vi "QR Reader.vi"() -> (0 "3":bool, 1 "2":bool, 2 "1":bool)   [LabVIEW 2017]
uses:
  <vilib>/vision/NI_Vision_Development_Module.lvlib
panel:
  out "index1":string
  out "QR_array":string[](array[string])
  out "Image Display":T1(plugin-control)
  in  "Stop (F)":bool
  out "Barcode Data":string
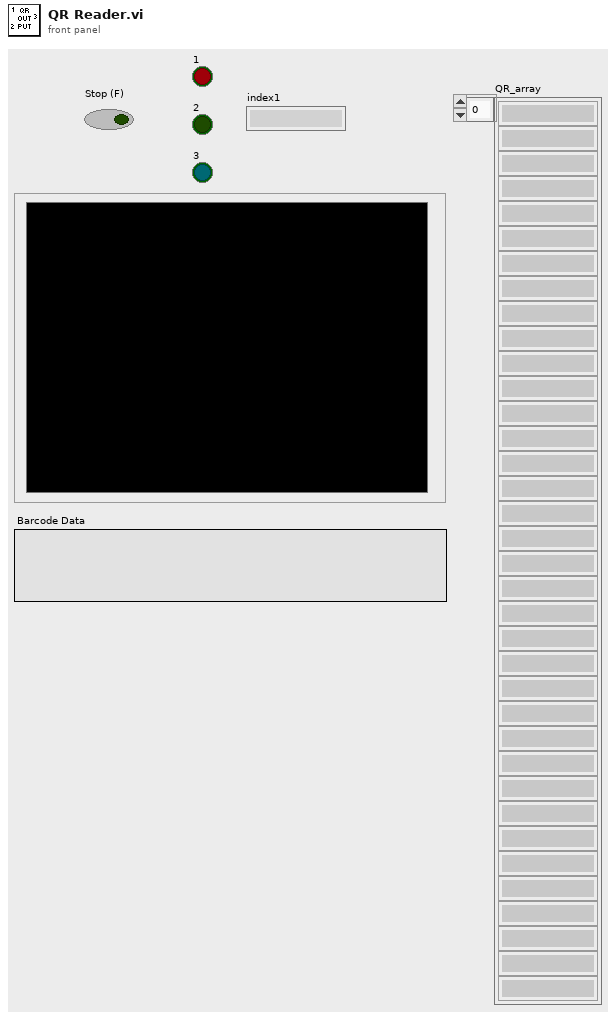
[diagram p1: front panel]
types:
  T1 = typedef "IMAQ Image.ctl" = refnum<image>
  T2 = typedef "QR Code Report.ctl" = cluster{"Found?":bool, "Data":string, "Bounding Box":cluster{"x":sgl, "y":sgl}[], "Errors Corrected":u32, "Dimensions (Rows/Cols)":u32, "Version":u32, "QR Model":T3, "Stream Mode":T4, "Barcode Polarity":T5, "Mirrored?":bool, "Append Stream Position":u32, "Size of Append Stream":u32, "First EAN-128 ID":i32, "First Alternate Language ID":i32, "Append Stream ID":u32, "Minimum Edge Strength":u32, "Demodulation Mode":T6, "Cell Sample Size":T7, "Cell Filter Mode":T8}
  T3 = typedef "QR Code Model Type.ctl" = i32
  T4 = typedef "QR Code Stream Mode Type.ctl" = i32
  T5 = typedef "Data Matrix Polarity.ctl" = i32
  T6 = typedef "Demodulation Mode.ctl" = i32
  T7 = typedef "Cell Sample Size.ctl" = i32
  T8 = typedef "Cell Filter Mode.ctl" = i32
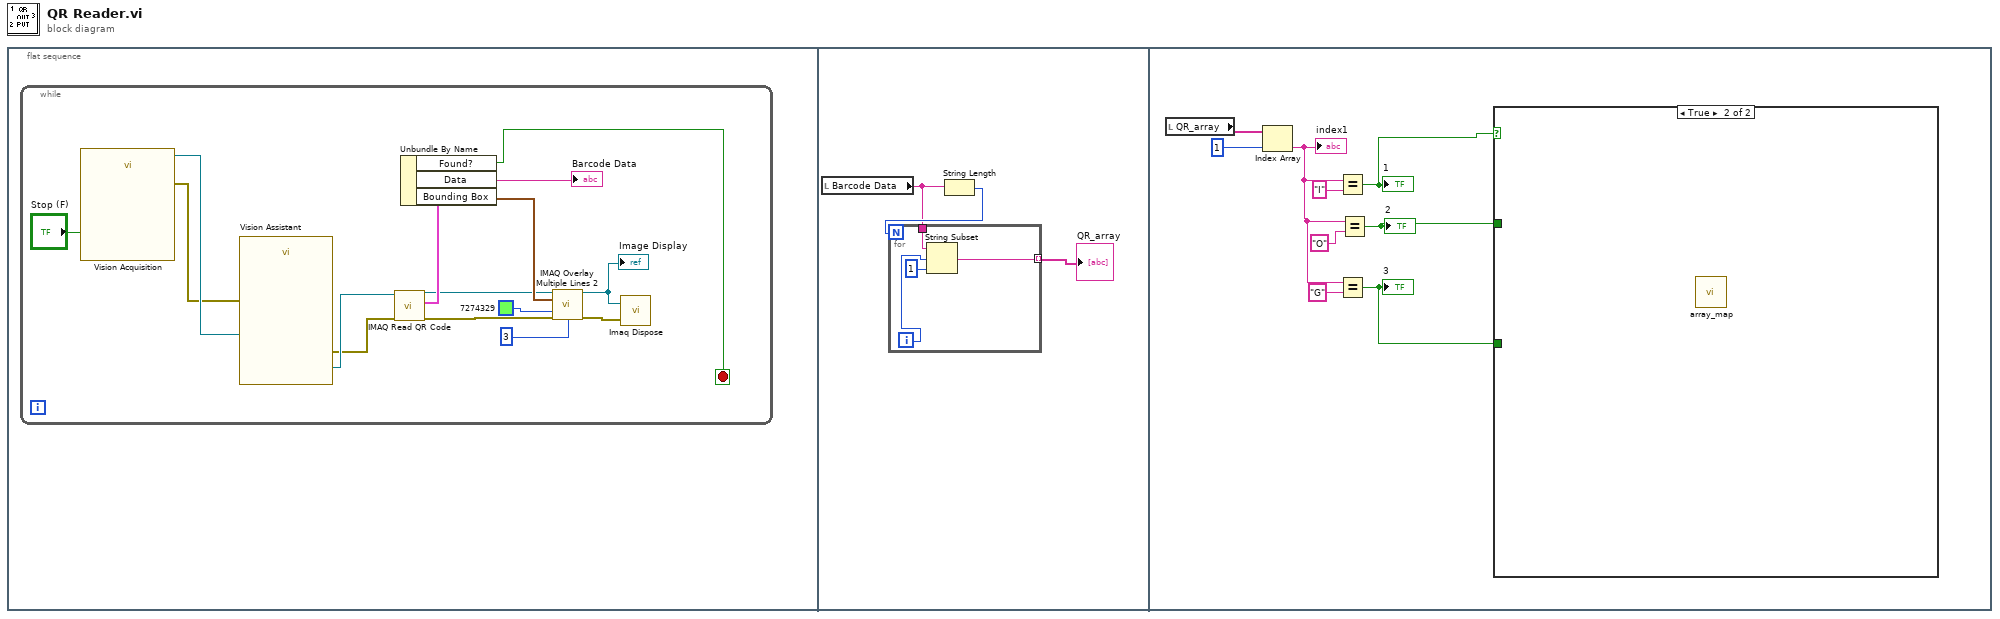
[diagram p0: block diagram]
diagram:
  n1 = flat-sequence {
    frame #0 {
      n2 = while {
        stop <- w8 stop-if-true
        n3 = call "Vision Acquisition"("Stop (F)"="Stop (F)") -> ("Image Out"=w13:T1, "error out"=w10:errorcluster)  [unwired: 24 in, 1 out]
        n4 = call "Vision Assistant"("Image In"=w13, "error in"=w10) -> ("Image Out"=w12:T1, "error out"=w11:errorcluster)  [unwired: 24 in]
        n5 = call "IMAQ Read QR Code"("error in (no error)"=w11, "Image"=w12) -> ("error out"=w2:errorcluster, "QR Code Report"=w14:T2, "Image (duplicate)"=w1:T1)  [unwired: 6 in, 1 out]
        n6 = Unbundle By Name(w14) -> ("Found?"=w8:bool, "Data"=→"Barcode Data":string, "Bounding Box"=w3:cluster{"x":sgl, "y":sgl}[])
        n7 = call "IMAQ Overlay Multiple Lines 2"("Image"=w1, "Line End Points"=w3, "Color"=u32 7274329, "error in (no error)"=w2, "Width"=u32 3) -> ("Image Out"=w7:T1, "error out"=w6:errorcluster)  [unwired: 9 in]
        "Image Display" <- w7
        n8 = call "Imaq Dispose"("Image"=w7, "error in (no error)"=w6) -> ()  [unwired: 4 in, 1 out]
      }
    }
    frame #1 {
      n9 = local read "Barcode Data"() -> (w17:string)
      n10 = String Length(string=w17) -> (length=w18:i32)
      n11 = for {
        N: w18 -> [_]
        tunnel: [w22] -> w16 mode=indexing
        tunnel: w17 -> [w21]
        i -> [w19]
        n12 = String Subset(string=w21, offset (0)=w19, length (rest)=1 ("length (rest)")) -> (substring=w22:string)
      }
      "QR_array" <- w16
    }
    frame #2 {
      n13 = local read "QR_array"() -> (w31:string[])
      n14 = Index Array(array=w31, index=1) -> (element=w27:string)
      "index1" <- w27
      n15 = Equal?(x=w27, y="I") -> (x = y?=w25:bool)
      "1" <- w25
      n16 = Equal?(x=w27, y="G") -> (x = y?=w23:bool)
      "3" <- w23
      n17 = Equal?(x=w27, y="O") -> (x = y?=w24:bool)
      "2" <- w24
      n18 = case shown="True" w25 {
        tunnel: w24 -> [w33 _]
        tunnel: w23 -> [w32 _]
        frame False {
          n19 = case shown="True" w33 {
            tunnel: w32 -> [w34 _]
            frame False {
              n20 = case shown="True" w34 {
                frame False {
                }
                frame True {
                }
              }
            }
            frame True {
            }
          }
        }
        frame True {
          n21 = call "array_map.vi"() -> ()  [unwired: 4 out]
        }
      }
    }
  }
